vi "DefaultFromIni.vi"(8 "error in (no error)":errorcluster, 11 "Sim_Ideal_PMU":refnum<class "Sim_Ideal_PMU.lvclass">) -> (0 "error out":errorcluster, 3 "Sim_Ideal_PMU":refnum<class "Sim_Ideal_PMU.lvclass">)   [LabVIEW 2018, in "SensorPlugins.lvlib" / "Sim_Ideal_PMU.lvclass"]
uses:
  Sim_Ideal_PMU.lvclass
  C:/Program Files (x86)/National Instruments/LabVIEW 2018/user.lib/NIST/BaseClasses/BasePlugin_class/BasePlugin.lvclass
  <userlib>/NIST/BaseClasses/BasePlugin_class/BasePlugin.lvclass/BasePlugin.ctl
  FGen/MemberClasses/FunctionBaseClass/FunctionBase.lvclass
  Sim_Ideal_PMU.lvclass/Sim_Ideal_PMU.ctl
  <userlib>/NIST/BaseClasses/BasePlugin_class/Accessors/Read PluginIniFilePath.vi
  Accessors/Write FunctionIniFilePath.vi
  Accessors/Write Function.vi
  <vilib>/Utility/error.llb/Error Cluster From Error Code.vi
  PmuBaseClass/PmuBase.lvclass
  <vilib>/ErrorRing/Error Ring.xnode
  <vilib>/Utility/config.llb/NI_LVConfig.lvlib
  <userlib>/NIST/BaseClasses/Object_class/BaseObject.lvclass
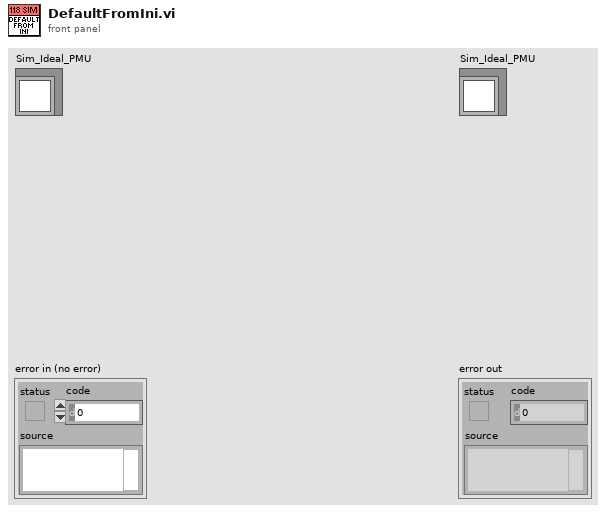
[diagram p1: front panel]
types:
  T1 = typedef "NI_LVConfig.lvlib/Config Data RefNum.ctl" = refnum<k1>
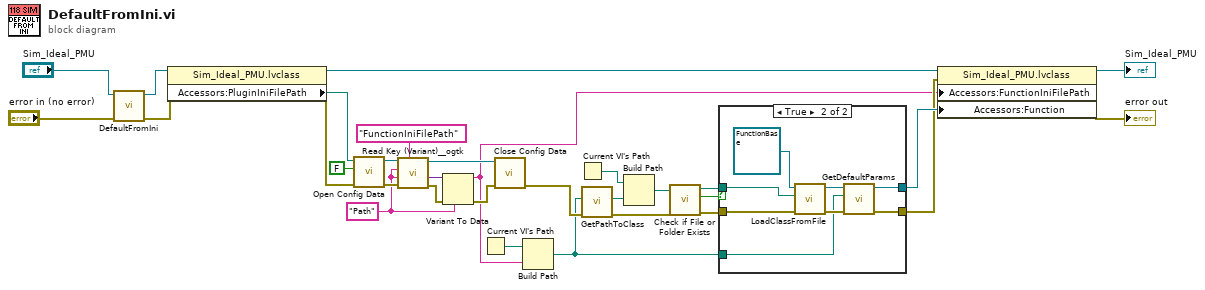
[diagram p0: block diagram]
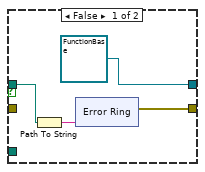
[diagram p2: hidden frame]
diagram:
  w18 = "Path" ("key (optional)")
  n1 = call-parent "DefaultFromIni.vi"("error in (no error)"="error in (no error)", "PmuBase in"="Sim_Ideal_PMU") -> ("error out"=w27:errorcluster, "PmuBase out"=w31:refnum<class "Sim_Ideal_PMU.lvclass">)  [unwired: 8 in]
  n2 = property class="Sim_Ideal_PMU.lvclass"(reference=w31, error in=w27) -> (reference out=w28:refnum<class "Sim_Ideal_PMU.lvclass">, error out=w25:errorcluster, "Accessors:PluginIniFilePath"=w26:path)
  n3 = call <vilib>:"Open Config Data.vi"("error in (no error)"=w25, "create file if necessary (T)"=FALSE, "configuration file path"=w26) -> ("error out"=w23:errorcluster, "refnum"=w2:T1)  [unwired: 6 in, 1 out]
  n4 = call <userlib>:"Read Key (Variant)__ogtk.vi"("section"="FunctionIniFilePath", "error in (no error)"=w23, "type"=w18, "key (optional)"=w18, "refnum"=w2) -> ("error out"=w21:errorcluster, "key-value"=w19:variant, "refnum out"=w17:T1)  [unwired: 3 in, 1 out]
  n5 = Variant To Data(error in=w21, type=w18, Variant=w19) -> (data=w1:string, error out=w16:errorcluster)
  n6 = Current VI's Path() -> (path=w7:path)
  n7 = call <vilib>:"Close Config Data.vi"("error in (no error)"=w16, "refnum"=w17) -> ("error out"=w15:errorcluster)  [unwired: 8 in, 1 out]
  n8 = Build Path(base path=w7, name or relative path=w1) -> (appended path=w6:path)
  n9 = Current VI's Path() -> (path=w14:path)
  n10 = call <userlib>:"GetPathToClass.vi"("error in (no error)"=w15, "configuration file path"=w6) -> ("error IO"=w11:errorcluster, "PathToClass"=w13:path)  [unwired: 8 in]
  n11 = Build Path(base path=w14, name or relative path=w13) -> (appended path=w12:path)
  n12 = call <vilib>:"Check if File or Folder Exists.vi"("error in (no error)"=w11, "path"=w12) -> ("error out"=w10:errorcluster, "file or folder exists?"=w8:bool, "dup path"=w9:path)  [unwired: 7 in]
  n13 = case shown="True" w8 {
    tunnel: [w34 w45] -> w4
    tunnel: w10 -> [_ w50]
    tunnel: w9 -> [w33 w49]
    tunnel: w6 -> [_ w43]
    tunnel: [refnum<class "FunctionBase.lvclass"> refnum ("Functions.lvlib:FunctionBase.lvclass") w44] -> w5
    frame False {
      n14 = Path To String(path=w33) -> (string=w35:string)
      n15 = xnode "Error Ring"("parameter 0"=w35) -> ("error out"=w34:errorcluster)
    }
    frame True {
      n16 = call-dynamic "LoadClassFromFile.vi"("error in (no error)"=w50, "class path"=w49, "reference in"=refnum<class "FunctionBase.lvclass"> refnum ("Functions.lvlib:FunctionBase.lvclass")) -> ("error out"=w47:errorcluster, "reference out"=w46:refnum<class "FunctionBase.lvclass">)  [unwired: 7 in]
      n17 = call-dynamic "GetDefaultParams.vi"("error in (no error)"=w47, "Path"=w43, "FunctionBase in"=w46) -> ("error out"=w45:errorcluster, "FunctionBase out"=w44:refnum<class "FunctionBase.lvclass">)  [unwired: 7 in]
    }
  }
  n18 = property class="Sim_Ideal_PMU.lvclass"(reference=w28, error in=w4, "Accessors:FunctionIniFilePath"=w1, "Accessors:Function"=w5) -> (reference out=→"Sim_Ideal_PMU":refnum<class "Sim_Ideal_PMU.lvclass">, error out=→"error out":errorcluster)
